vi "ReadCapacitanceBuffers.vi"(8 "error in (no error)":errorcluster, 10 "Status":refnum<vi>, 11 "VISA Refnum in":refnum<visa-resource-name>) -> (0 "error out":errorcluster, 3 "CapacitanceInfos":T1[](array[typedef]))   [LabVIEW 2020]
uses:
  CapacitanceRecord.ctl
  Keithley 2600 Series/Keithley 2600 Series.lvlib
panel:
  out "Array":string[](array[string])
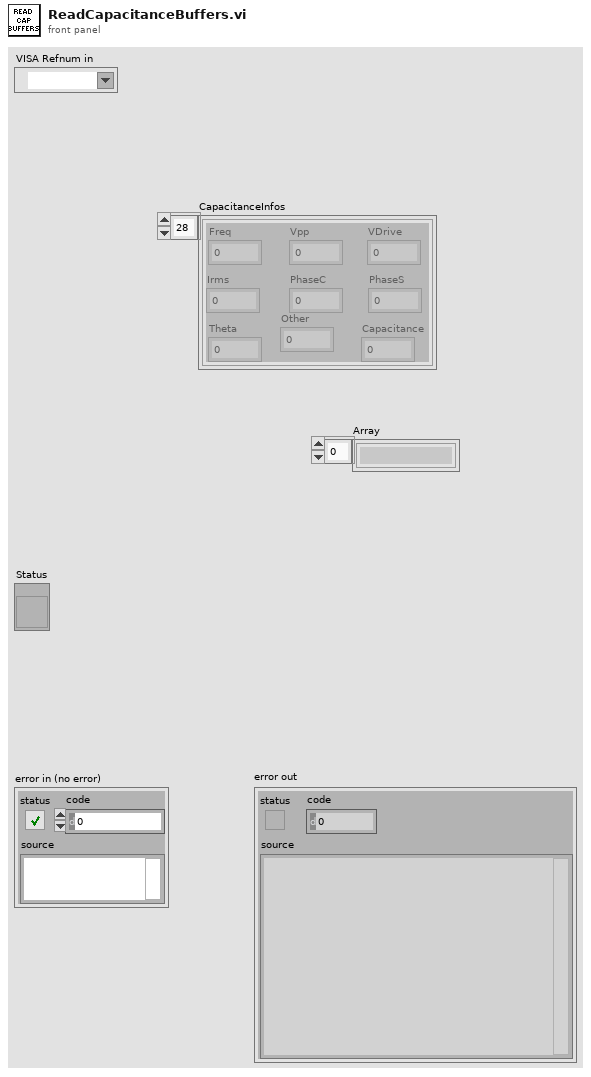
[diagram p1: front panel]
types:
  T1 = typedef "CapacitanceRecord.ctl" = cluster{"Freq":dbl, "Vpp":dbl, "PhaseS":dbl, "Irms":dbl, "PhaseC":dbl, "Theta":dbl, "VDrive":dbl, "Capacitance":dbl, "Other":dbl}
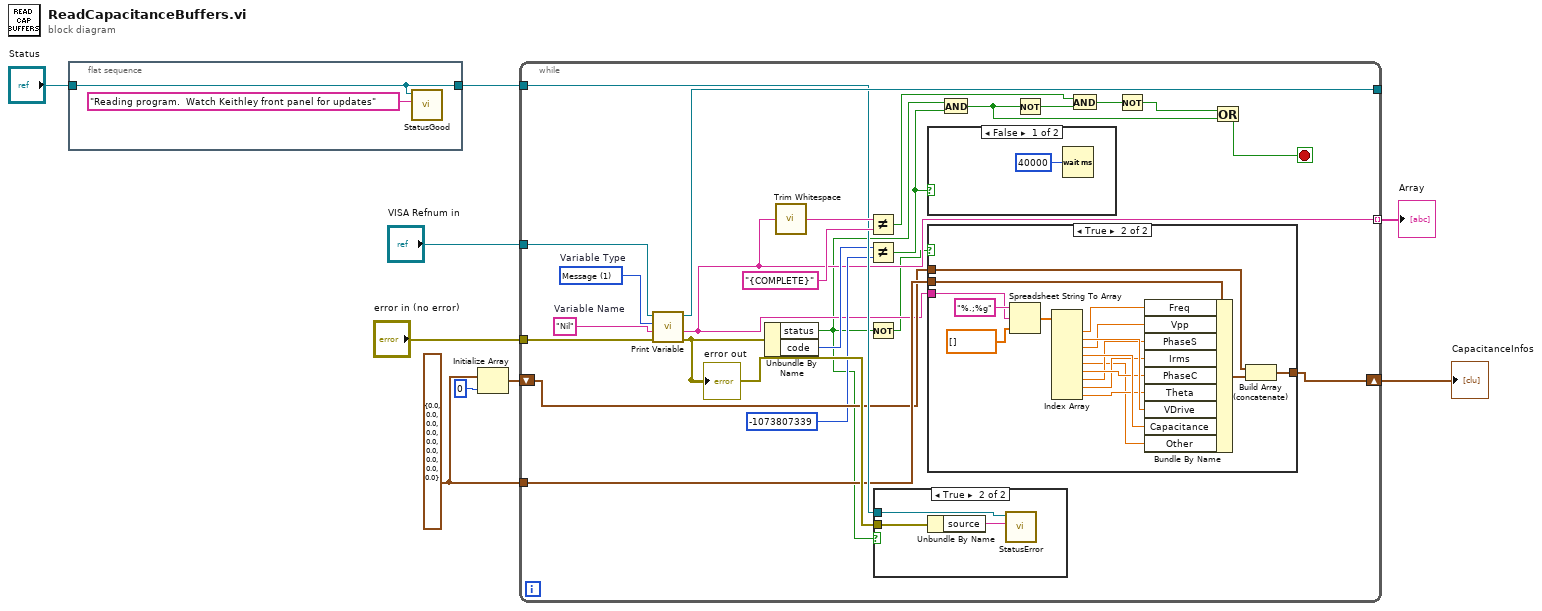
[diagram p0: block diagram]
diagram:
  w5 = T1 {"Freq"=0.0, "Vpp"=0.0, "PhaseS"=0.0, "Irms"=0.0, "PhaseC"=0.0, "Theta"=0.0, "VDrive"=0.0, "Capacitance"=0.0, "Other"=0.0} ("cluster")
  n1 = flat-sequence {
    tunnel: "Status" -> [w10]
    tunnel: [w10] -> w1
    frame #0 {
      n2 = call "StatusGood.vi"("Text.Text"="Reading program.  Watch Keithley front panel for updates", "String in"=w10) -> ()  [unwired: 10 in]
    }
  }
  n3 = Initialize Array(w5, 0 ("dimension size")) -> (w4:T1[])
  n4 = while {
    tunnel: "VISA Refnum in" -> [w14]
    tunnel: "error in (no error)" -> [w13]
    tunnel: [w33] -> _
    shift-right: [w25] -> w6
    shift-left: w4 -> [w23]
    tunnel: w1 -> [w26]
    tunnel: w5 -> [w24]
    tunnel: [w17] -> w3 mode=indexing
    stop <- w28 stop-if-true
    w35 = 1 items=["Number", "Message"]  # Variable Type
    w34 = "Nil"  # Variable Name
    n5 = call "Print Variable.vi"("error in (no error)"=w13, "Variable Name"=w34, "Variable Type (0: Number)"=w35, "VISA resource name"=w14) -> ("error out"=w27:errorcluster, "Message"=w17:string, "VISA resource name out"=w33:refnum<visa-resource-name>)  [unwired: 4 in, 1 out]
    "error out" <- w27
    n6 = Unbundle By Name(w27) -> ("status"=w16:bool, "code"=w22:i32)
    n7 = call <vilib>:"Trim Whitespace.vi"("string"=w17) -> ("trimmed string"=w32:string)  [unwired: 1 in]
    n8 = Not Equal?(x=w32, y="{COMPLETE}") -> (x != y?=w30:bool)
    n9 = Not Equal?(x=w22, y=-1073807339) -> (x != y?=w12:bool)
    n10 = Not(x=w16) -> (.not. x?=w15:bool)
    n11 = case shown="True" w16 {
      tunnel: w27 -> [_ w38]
      tunnel: w26 -> [_ w37]
      frame False {
      }
      frame True {
        n12 = Unbundle By Name(w38) -> ("source"=w39:string)
        n13 = call "StatusError.vi"("Text.Text"=w39, "String in"=w37) -> ()  [unwired: 10 in]
      }
    }
    n14 = case shown="False" w12 {
      frame False {
        n15 = Wait (ms)(milliseconds to wait=u32 40000) -> ()  [unwired: 1 out]
      }
      frame True {
      }
    }
    n16 = case shown="True" w15 {
      tunnel: w17 -> [_ w55]
      tunnel: w23 -> [w40 w54]
      tunnel: [w40 w53] -> w25
      tunnel: w24 -> [_ w52]
      frame False {
      }
      frame True {
        n17 = Spreadsheet String To Array(format string="%.;%g", spreadsheet string=w55, array type (2D Dbl)=dbl[] []) -> (array=w50:dbl[])  [unwired: 1 in]
        n18 = Index Array(array=w50) -> (element #1=w49:dbl, element #2=w48:dbl, element #3=w47:dbl, element #4=w46:dbl, element #5=w41:dbl, element #6=w45:dbl, element #7=w44:dbl, element #8=w43:dbl, element #9=w42:dbl)  [unwired: 9 in]
        n19 = Bundle By Name(cluster=w52, "Freq"=w49, "Vpp"=w47, "PhaseS"=w44, "Irms"=w43, "PhaseC"=w45, "Theta"=w42, "VDrive"=w48, "Capacitance"=w46, "Other"=w41) -> (w51:T1)
        n20 = Build Array (concatenate)(w54, w51) -> (w53:T1[])
      }
    }
    n21 = And(x=w16, y=w12) -> (x .and. y?=w19:bool)
    n22 = Not(x=w19) -> (.not. x?=w18:bool)
    n23 = And(x=w30, y=w18) -> (x .and. y?=w20:bool)
    n24 = Not(x=w20) -> (.not. x?=w29:bool)
    n25 = Or(x=w29, y=w19) -> (x .or. y?=w28:bool)
  }
  "CapacitanceInfos" <- w6
  "Array" <- w3
